vi "SetLogFormatter.vi"(8 "Error in (no error)":errorcluster, 10 "LogFormatterInterface in":refnum<class "LogFormatterInterface.lvclass">, 11 "LogWriterInterface in":refnum<class "LogWriterInterface.lvclass">) -> (0 "Error out":errorcluster, 3 "LogWriterInterface out":refnum<class "LogWriterInterface.lvclass">)   [LabVIEW 2011, in "LogWriterInterface.lvclass"]
uses:
  LogWriterInterface.lvclass
  Formatter/LogFormatterInterface/LogFormatterInterface.lvclass
  LogWriterInterface.lvclass/LogWriterInterface.ctl
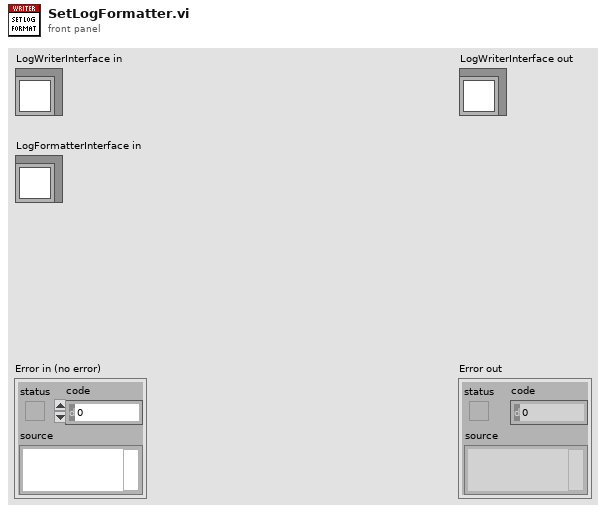
[diagram p1: front panel]
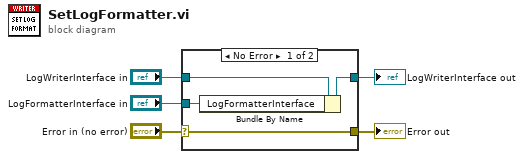
[diagram p0: block diagram]
diagram:
  n1 = case shown="No Error" "Error in (no error)" {
    selector: "Error in (no error)" -> [w9 w10]
    tunnel: [w9 w10] -> w4
    tunnel: [w7 w11] -> w2
    tunnel: "LogWriterInterface in" -> [w8 w11]
    tunnel: "LogFormatterInterface in" -> [w6 _]
    frame No Error {
      n2 = Bundle By Name(cluster=w8, "LogFormatterInterface"=w6) -> (w7:refnum<class "LogWriterInterface.lvclass">)
    }
    frame Error {
    }
  }
  "Error out" <- w4
  "LogWriterInterface out" <- w2
